vi "DAQmx Read (Digital 1D Bool 1Chan 1Samp).vi"(0 "task/channels in":refnum<k21>, 9 "timeout":dbl=10.0 format="%0.2f", 11 "error in":errorcluster) -> (4 "task out":refnum<k21>, 6 "data":bool[](array[boolean]), 15 "error out":errorcluster)   [LabVIEW 2017]
doc: "Reads an array of Boolean values from a task that contains a single digital input channel."
uses:
  nilvaiu.dll
panel:
  # "line"
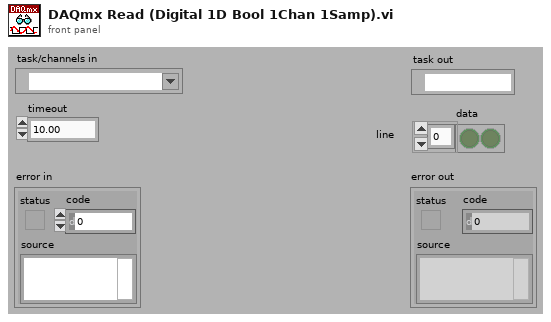
[diagram p1: front panel]
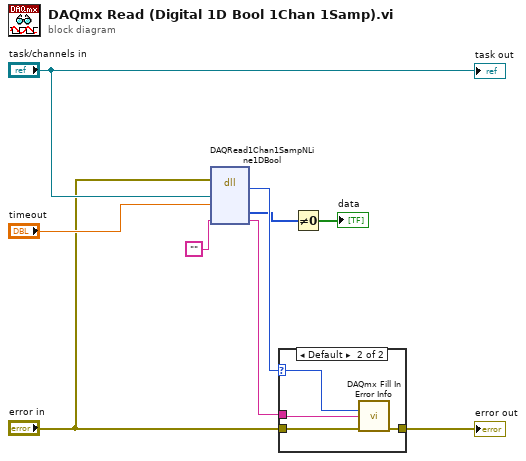
[diagram p0: block diagram]
diagram:
  n1 = dll-call lib="nilvaiu.*" fn="DAQRead1Chan1SampNLine1DBool"(error in="error in", "taskID"="task/channels in", "timeout"="timeout", "extendedErrorInfo"="") -> ("return type"=w7:i32, "data"=w5:u8[], "extendedErrorInfo"=w4:string)  [unwired: 4 in, 3 out]
  n2 = case shown="Default" w7 {
    selector: w7 -> [_ w13]
    tunnel: "error in" -> [w10 w14]
    tunnel: [w10 w12] -> w9
    tunnel: w4 -> [_ w11]
    frame 0 {
    }
    frame Default {
      n3 = call "DAQmx Fill In Error Info.vi"("status code"=w13, "extended error info"=w11, "error in"=w14) -> ("error out"=w12:errorcluster)  [unwired: 1 in, 11 out]
    }
  }
  "error out" <- w9
  n4 = Not Equal To 0?(x=w5) -> (x != 0?=→"data":bool[])
  "task out" <- "task/channels in"
